vi "getCurrentCVTVals.vi"(8 "error in":errorcluster, 11 "channel number":i32) -> (0 "error out":errorcluster, 2 "speed":dbl, 3 "position":dbl)   [LabVIEW 2020]
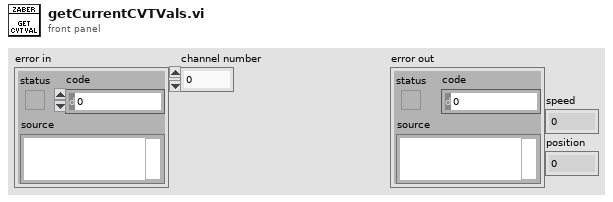
[diagram p1: front panel]
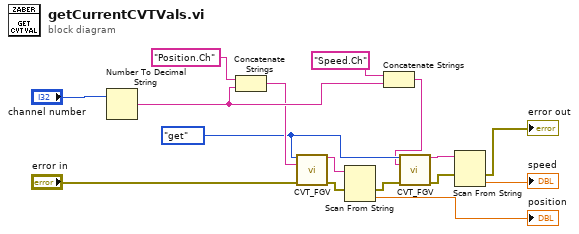
[diagram p0: block diagram]
diagram:
  w12 = enum16{"set", "get", "reset", "get all"}."get" ("command")
  n1 = Number To Decimal String(number="channel number") -> (decimal integer string=w16:string)  [unwired: 1 in]
  n2 = Concatenate Strings("Position.Ch" ("command or variable name"), w16) -> (w13:string)
  n3 = call "CVT_FGV.vi"("command"=w12, "variable"=w13, "error in"="error in") -> ("value out"=w4:string, "error out"=w3:errorcluster)  [unwired: 10 in, 1 out]
  n4 = Scan From String(input string=w4, error in=w3) -> (error out=w2:errorcluster, output 1=→"position":dbl)  [unwired: 3 in, 2 out]
  n5 = Concatenate Strings("Speed.Ch" ("command or variable name"), w16) -> (w9:string)
  n6 = call "CVT_FGV.vi"("command"=w12, "variable"=w9, "error in"=w2) -> ("value out"=w8:string, "error out"=w7:errorcluster)  [unwired: 10 in, 1 out]
  n7 = Scan From String(input string=w8, error in=w7) -> (error out=→"error out":errorcluster, output 1=→"speed":dbl)  [unwired: 3 in, 2 out]
